vi "Build Hex Command String.vi"(6 "Length":string="\b", 7 "Data (Dec)":string="\u0004", 8 "Error In":errorcluster, 11 "Command (Hex)":string="\u0001") -> (0 "Error Out":errorcluster, 2 "Command String":string)   [LabVIEW 2018, in "Hitronics.lvlib" / "Hitronics.lvclass"]
uses:
  Hitronics.lvclass
panel:
  out "Checksum":string
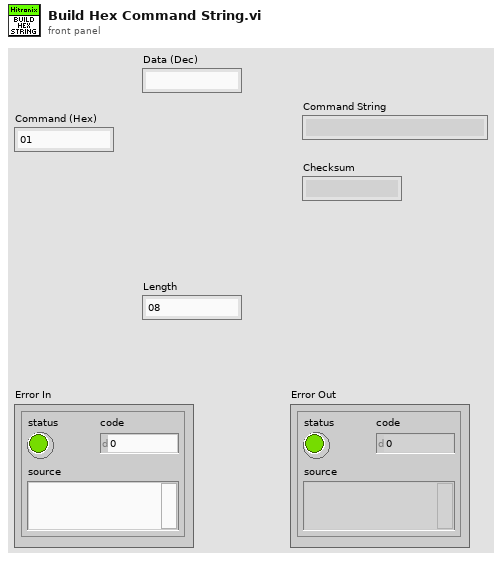
[diagram p1: front panel]
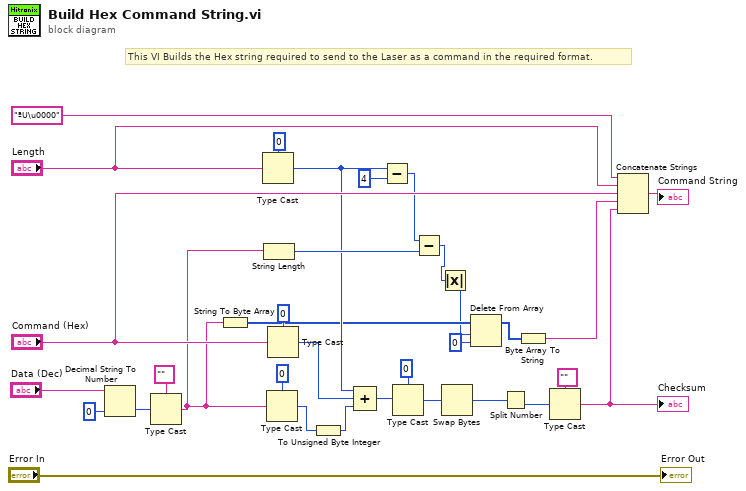
[diagram p0: block diagram]
diagram:
  # "This VI Builds the Hex string required to send to the Laser as a command in the required format."
  n1 = Decimal String To Number(string="Data (Dec)", default (0L)=0 ("default (0 I32)")) -> (number=w11:i32)  [unwired: 1 in, 1 out]
  n2 = Type Cast(type="" ("hex integer string"), x=w11) -> (*(type *) &x=w8:string)
  n3 = String To Byte Array(string=w8) -> (unsigned byte array=w7:u8[])
  n4 = Type Cast(type=u8 0, x="Length") -> (*(type *) &x=w18:u8)
  n5 = String Length(string=w8) -> (length=w20:i32)
  n6 = Type Cast(type=0, x=w8) -> (*(type *) &x=w14:i32)
  n7 = Type Cast(type=u8 0, x="Command (Hex)") -> (*(type *) &x=w31:u8)
  n8 = To Unsigned Byte Integer(number=w14) -> (unsigned 8bit integer=w13:u8)
  n9 = Compound Arithmetic op=ADD(w18, w31, w13) -> (w30:u8)
  n10 = Subtract(x=w18, y=u8 4) -> (x-y=w21:u8)
  n11 = Type Cast(type=u16 0 ("*(type *) &x 5"), x=w30) -> (*(type *) &x=w28:u16)
  n12 = Subtract(x=w21, y=w20) -> (x-y=w6:i32)
  n13 = Absolute Value(x=w6) -> (abs(x)=w5:i32)
  n14 = Swap Bytes(anything=w28) -> (byte swapped=w26:u16)
  n15 = Delete From Array(array=w7, length=w5, index=0) -> (array with subset deleted=w4:u8[])  [unwired: 1 out]
  n16 = Split Number(x=w26) -> (lo(x)=w22:u8)  [unwired: 1 out]
  n17 = Byte Array To String(unsigned byte array=w4) -> (string=w2:string)
  n18 = Type Cast(type="" ("Command"), x=w22) -> (*(type *) &x=w1:string)
  "Checksum" <- w1
  n19 = Concatenate Strings("ªU\u0000" ("string"), "Length", "Command (Hex)", w2, w1) -> (→"Command String":string)
  "Error Out" <- "Error In"
